vi "RMS.vi"(7 "SlaveID":u8=1, 8 "error in (no error)":errorcluster, 11 ".NET Refnum in":refnum<k24>) -> (0 "error out":errorcluster, 2 "OA":u16[][](array[numeric]), 3 "reference out":refnum<k24>)   [LabVIEW 2017]
uses:
  C:/Users/chrisjan/Desktop/NowWorking/ITRI/DLL/Modbus.dll
  DLL/Modbus.dll
panel:
  out "x-y":u32
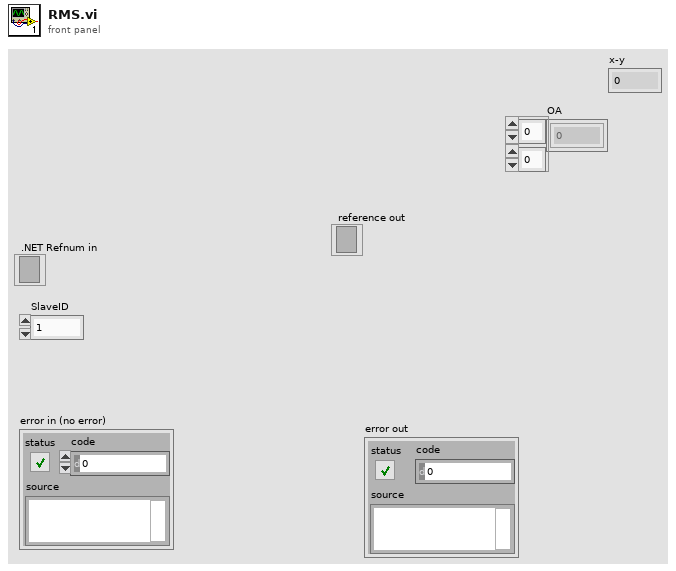
[diagram p1: front panel]
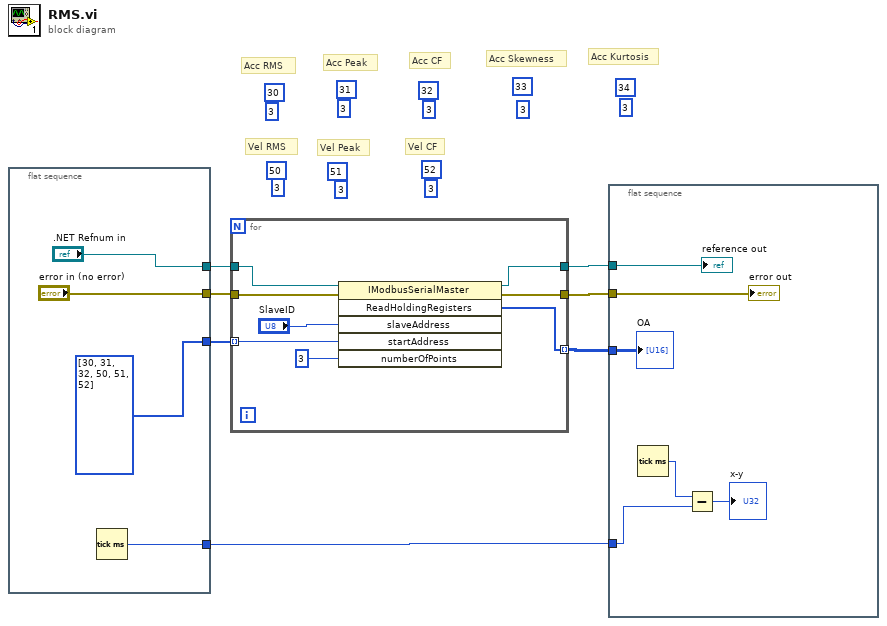
[diagram p0: block diagram]
diagram:
  (unwired) u16 3 ("numberOfPoints")
  (unwired) u16 3 ("numberOfPoints")
  (unwired) u16 52 ("startAddress")
  (unwired) u16 51 ("startAddress")
  (unwired) u16 3 ("numberOfPoints")
  (unwired) u16 3 ("numberOfPoints")
  (unwired) u16 3 ("numberOfPoints")
  (unwired) u16 50 ("startAddress")
  (unwired) u16 34 ("startAddress")
  (unwired) u16 33 ("startAddress")
  (unwired) u16 3 ("numberOfPoints")
  (unwired) u16 32 ("startAddress")
  (unwired) u16 3 ("numberOfPoints")
  (unwired) u16 31 ("startAddress")
  (unwired) u16 3 ("numberOfPoints")
  (unwired) u16 30 ("startAddress")
  # "Vel CF"
  # "Vel Peak"
  # "Vel RMS"
  # "Acc Kurtosis"
  # "Acc Skewness"
  # "Acc CF"
  # "Acc Peak"
  # "Acc RMS"
  n1 = flat-sequence {
    tunnel: ["error in (no error)"] -> w7
    tunnel: [".NET Refnum in"] -> w6
    tunnel: [u16[] [30, 31, 32, 50, 51, 52]] -> w3
    tunnel: [w8] -> w1
    frame #0 {
      n2 = Tick Count (ms)() -> (millisecond timer value=w8:u32)
    }
  }
  n3 = for {
    tunnel: w7 -> [w18]
    tunnel: [w16] -> w5
    tunnel: w3 -> [w13] mode=indexing
    tunnel: [w12] -> w2 mode=indexing
    tunnel: w6 -> [w17]
    tunnel: [w15] -> w4
    n4 = invoke class="IModbusSerialMaster" method="ReadHoldingRegisters"(reference=w17, error in=w18, "slaveAddress"="SlaveID", "startAddress"=w13, "numberOfPoints"=u16 3) -> (reference out=w15:refnum<k24>, error out=w16:errorcluster, "ReadHoldingRegisters"=w12:u16[])  [unwired: 1 in, 3 out]
  }
  n5 = flat-sequence {
    tunnel: w5 -> [w25]
    tunnel: w4 -> [w24]
    tunnel: w2 -> [w23]
    tunnel: w1 -> [w21]
    frame #0 {
      n6 = Tick Count (ms)() -> (millisecond timer value=w22:u32)
      n7 = Subtract(x=w22, y=w21) -> (x-y=→"x-y":u32)
      "error out" <- w25
      "reference out" <- w24
      "OA" <- w23
    }
  }
